vi "Update thickness.vi"(8 "error in (no error)":errorcluster, 10 "Thickness":string, 11 "Stack in":refnum<class "Stack.lvclass">) -> (0 "error out":errorcluster, 3 "Stack out":refnum<class "Stack.lvclass">)   [LabVIEW 2021, in "Stack.lvclass"]
uses:
  Stack.lvclass
  Stack.lvclass/Stack.ctl
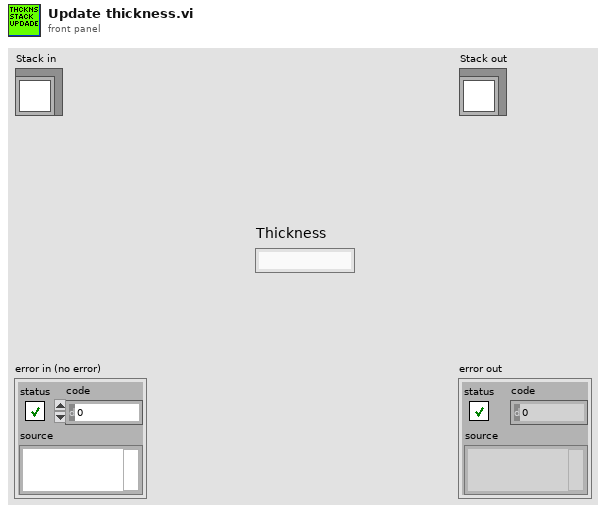
[diagram p1: front panel]
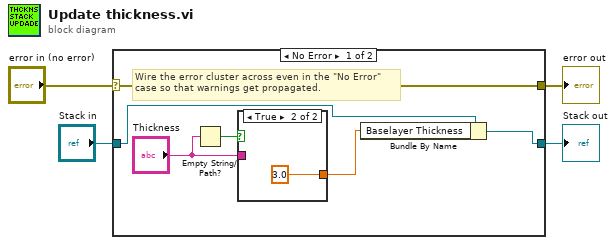
[diagram p0: block diagram]
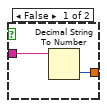
[diagram p2: hidden frame]
diagram:
  n1 = case shown="No Error" "error in (no error)" {
    selector: "error in (no error)" -> [w10 w15]
    tunnel: [w10 w15] -> w3
    tunnel: [w8 w14] -> w1
    tunnel: "Stack in" -> [w9 w14]
    frame No Error {
      # "Wire the error cluster across even in the \"No Error\"\ncase so that warnings get propagated."
      n2 = Empty String/Path?(string/path="Thickness") -> (empty?=w5:bool)
      n3 = case shown="True" w5 {
        tunnel: [w12 3.0] -> w7
        tunnel: "Thickness" -> [w11 _]
        frame False {
          n4 = Decimal String To Number(string=w11) -> (number=w12:i32)  [unwired: 2 in, 1 out]
        }
        frame True {
        }
      }
      n5 = Bundle By Name(cluster=w9, "Baselayer Thickness"=w7) -> (w8:refnum<class "Stack.lvclass">)
    }
    frame Error {
    }
  }
  "error out" <- w3
  "Stack out" <- w1
